vi "Concatenate Waveform Array.vi"(0 "waveform array":waveform(dbl)[](array[waveform])) -> (4 "waveform t0 array":dbl[](array[numeric]), 6 "waveform dt array":dbl[](array[numeric]), 8 "waveform length array":i32[](array[numeric]), 10 "concatenated waveform Y":dbl[](array[numeric]))   [LabVIEW 2021, in "PMIC Common.lvlib"]
uses:
  PMIC Common.lvlib
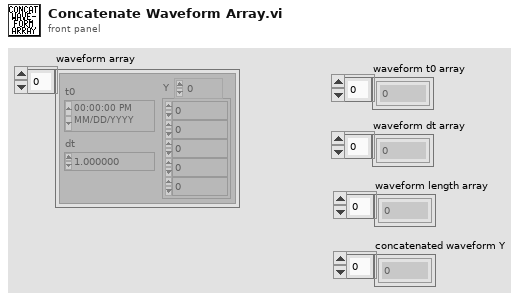
[diagram p1: front panel]
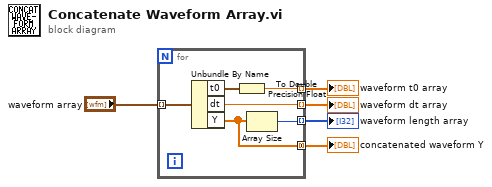
[diagram p0: block diagram]
diagram:
  n1 = for {
    tunnel: "waveform array" -> [w11] mode=indexing
    tunnel: [w9] -> w3 mode=indexing
    tunnel: [w8] -> w4 mode=indexing
    tunnel: [w7] -> w2 mode=indexing
    tunnel: [w6] -> w1 mode=concatenating
    n2 = Unbundle By Name(w11) -> ("t0"=w10:timestamp, "dt"=w9:dbl, "Y"=w6:dbl[])
    n3 = To Double Precision Float(number=w10) -> (double precision float=w8:dbl)
    n4 = Array Size(array=w6) -> (size(s)=w7:i32)
  }
  "waveform t0 array" <- w4
  "waveform dt array" <- w3
  "waveform length array" <- w2
  "concatenated waveform Y" <- w1
